vi "GetEnumFeatureEntryNum.vi"(9 "handle":i64, 10 "pFeatureName":string, 11 "error in (no error)":errorcluster) -> (2 "pEntryNum":u32, 3 "error out":errorcluster)   [LabVIEW 2016]
uses:
  MVSDKmd.dll
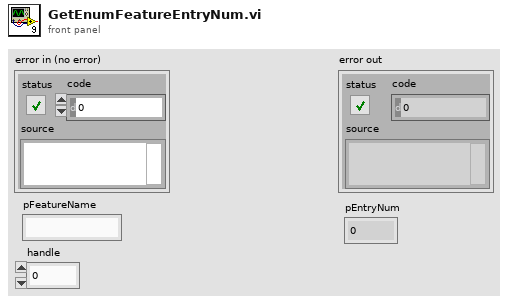
[diagram p1: front panel]
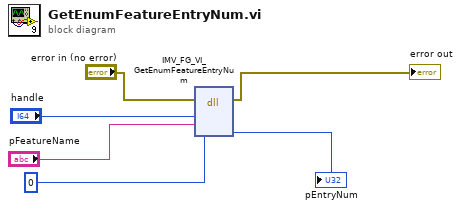
[diagram p0: block diagram]
diagram:
  n1 = dll-call lib="MVSDKmd.dll" fn="IMV_FG_VI_GetEnumFeatureEntryNum"(error in="error in (no error)", "handle"="handle", "pFeatureName"="pFeatureName", "pEntryNum"=u32 0) -> (error out=→"error out":errorcluster, "pEntryNum"=→"pEntryNum":u32)  [unwired: 5 in, 1 out]
